vi "get channels.vi"(11 "Simple Sequencer TBM configuration in":refnum<class "Simple Sequencer TBM configuration.lvclass">) -> (2 "channels":refnum<class "TBM channel.lvclass">[](array[class]), 3 "Simple Sequencer TBM configuration out":refnum<class "Simple Sequencer TBM configuration.lvclass">)   [LabVIEW 2014, in "Simple Sequencer TBM configuration.lvclass"]
doc: "Returns a list of channels configured for the sequencer."
uses:
  Simple Sequencer TBM configuration.lvclass
  <vilib>/NI/Tag Bus Module Framework/channel/TBM channel.lvclass
  sequencer parent classes/sequencer config parent/base TBM sequencer configuration.lvclass
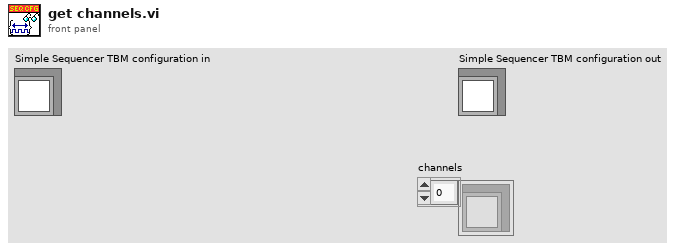
[diagram p1: front panel]
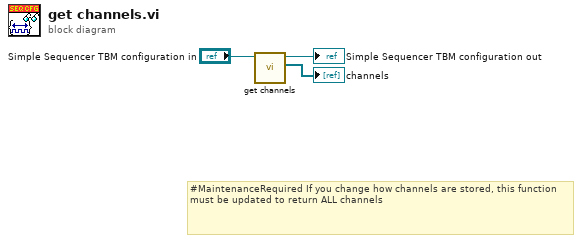
[diagram p0: block diagram]
diagram:
  # "#MaintenanceRequired If you change how channels are stored, this function must be updated to return ALL channels"
  n1 = call-parent "get channels.vi"("module configuration in"="Simple Sequencer TBM configuration in") -> ("channels"=→"channels":refnum<class "TBM channel.lvclass">[], "module configuration out"=→"Simple Sequencer TBM configuration out":refnum<class "Simple Sequencer TBM configuration.lvclass">)  [unwired: 9 in]
